vi "execCommand.vi"(8 "error in (no error)":errorcluster, 9 "context":refnum<class "Context.lvclass">, 10 "command":refnum<class "Command.lvclass">, 11 "InvokerThisContext in":refnum<class "InvokerThisComponent.lvclass">) -> (0 "error out":errorcluster, 1 "context 2":refnum<class "Context.lvclass">, 3 "InvokerThisContext out":refnum<class "InvokerThisComponent.lvclass">)   [LabVIEW 2015, in "InvokerThisComponent.lvclass"]
doc: "Executes the received command dynamically."
uses:
  InvokerThisComponent.lvclass
  ComponentTemplateCore/ComponentModel/ComponentModel/Command/Command.lvclass
  ComponentTemplateCore/ComponentModel/ComponentModel/Context/Context.lvclass
  CommandThisComponent/CommandThisComponent.lvclass
  IContextThisComponent/IContextThisComponent.lvclass
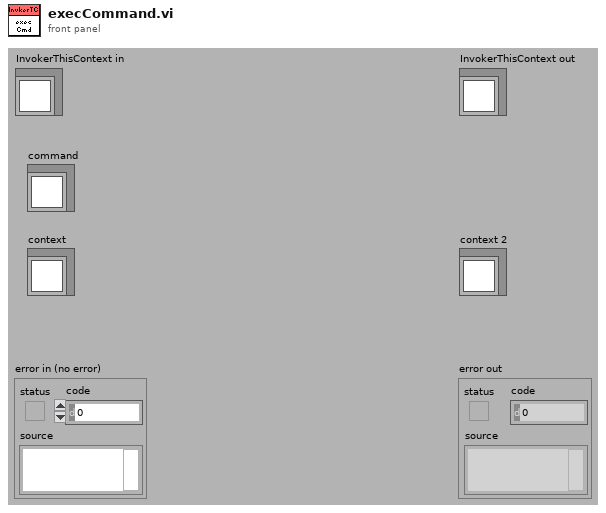
[diagram p1: front panel]
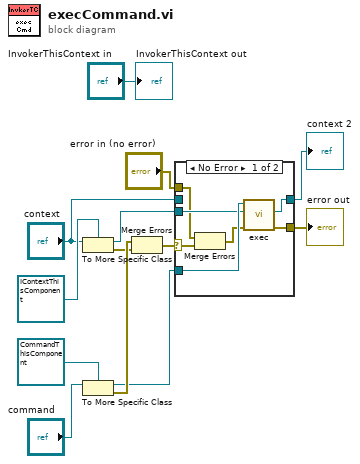
[diagram p0: block diagram]
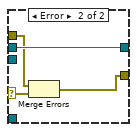
[diagram p2: hidden frame]
diagram:
  n1 = To More Specific Class(target class=refnum<class "IContextThisComponent.lvclass"> refnum ("ContextThisComponent.lvlib:ContextThisComponent.lvclass"), reference="context") -> (specific class reference=w5:refnum<class "IContextThisComponent.lvclass">, error out=w8:errorcluster)  [unwired: 1 in]
  n2 = To More Specific Class(target class=refnum<class "CommandThisComponent.lvclass"> refnum ("CommandThisComponent.lvlib:CommandThisComponent.lvclass"), reference="command") -> (specific class reference=w6:refnum<class "CommandThisComponent.lvclass">, error out=w9:errorcluster)  [unwired: 1 in]
  n3 = Merge Errors(w9, w8) -> (w7:errorcluster)
  n4 = case shown="No Error" w7 {
    selector: w7 -> [w16 w21]
    tunnel: w6 -> [w20 _]
    tunnel: w5 -> [w19 _]
    tunnel: [w18 w23] -> w2
    tunnel: [w17 w24] -> w4
    tunnel: "context" -> [_ w24]
    tunnel: "error in (no error)" -> [w15 w22]
    frame No Error {
      n5 = Merge Errors(w15, w16) -> (w14:errorcluster)
      n6 = call-dynamic "exec.vi"("error in (no error)"=w14, "context"=w19, "Command in"=w20) -> ("error out"=w18:errorcluster, "context 2"=w17:refnum<class "IContextThisComponent.lvclass">)  [unwired: 6 in, 1 out]
    }
    frame Error {
      n7 = Merge Errors(w22, w21) -> (w23:errorcluster)
    }
  }
  "error out" <- w2
  "context 2" <- w4
  "InvokerThisContext out" <- "InvokerThisContext in"
